vi "Process.vi"(8 "error in":errorcluster, 11 "Plugin in":refnum<class "Sift Stream.lvclass">) -> (0 "error out":errorcluster, 3 "Plugin out":refnum<class "Sift Stream.lvclass">)   [LabVIEW 2024, in "Sift Stream.lvlib" / "Sift Stream.lvclass"]
uses:
  Sift Stream.lvclass
  Sift Stream.lvclass/Sift Stream.ctl
  <vilib>/Utility/error.llb/Error Cluster From Error Code.vi
  <vilib>/ErrorRing/Error Ring.xnode
  <vilib>/Sift/Sift/Sift API/Sift Client.lvclass
  <vilib>/FlexLogger/SDK/PluginSDK.lvlibp/PEFClasses/SDK/Plugin/Plugin.lvclass
  <vilib>/Sift/Sift/Sift Client.lvlib
  C:/Program Files/National Instruments/LabVIEW 2024/vi.lib/FlexLogger/SDK/PluginSDK.lvlibp/PEFClasses/SDK/Plugin/Plugin.lvclass
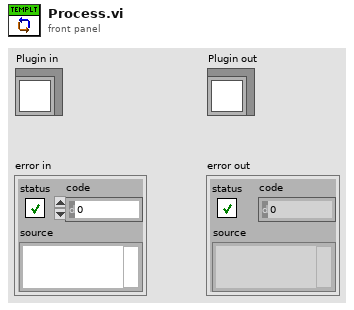
[diagram p1: front panel]
types:
  T1 = typedef "Sift Client.lvlib/Timestamp.ctl" = cluster{"seconds":i64, "nanos":i32}
  T2 = cluster{"Channel Setpoints":dbl[], "Names":string[]}
  T3 = typedef "Sift Stream.lvlib/Sift Stream.lvclass/Sift Stream Parameters.ctl" = cluster{"API gRPC URL":string, "API REST URL":string, "API Key":string, "Asset Name":string, "Data Rate":dbl, "Stream Names":string[], "Sift Client":refnum<class "Sift Client.lvclass">, "Session Error":errorcluster, "Stop Notifier":refnum<notifier>}
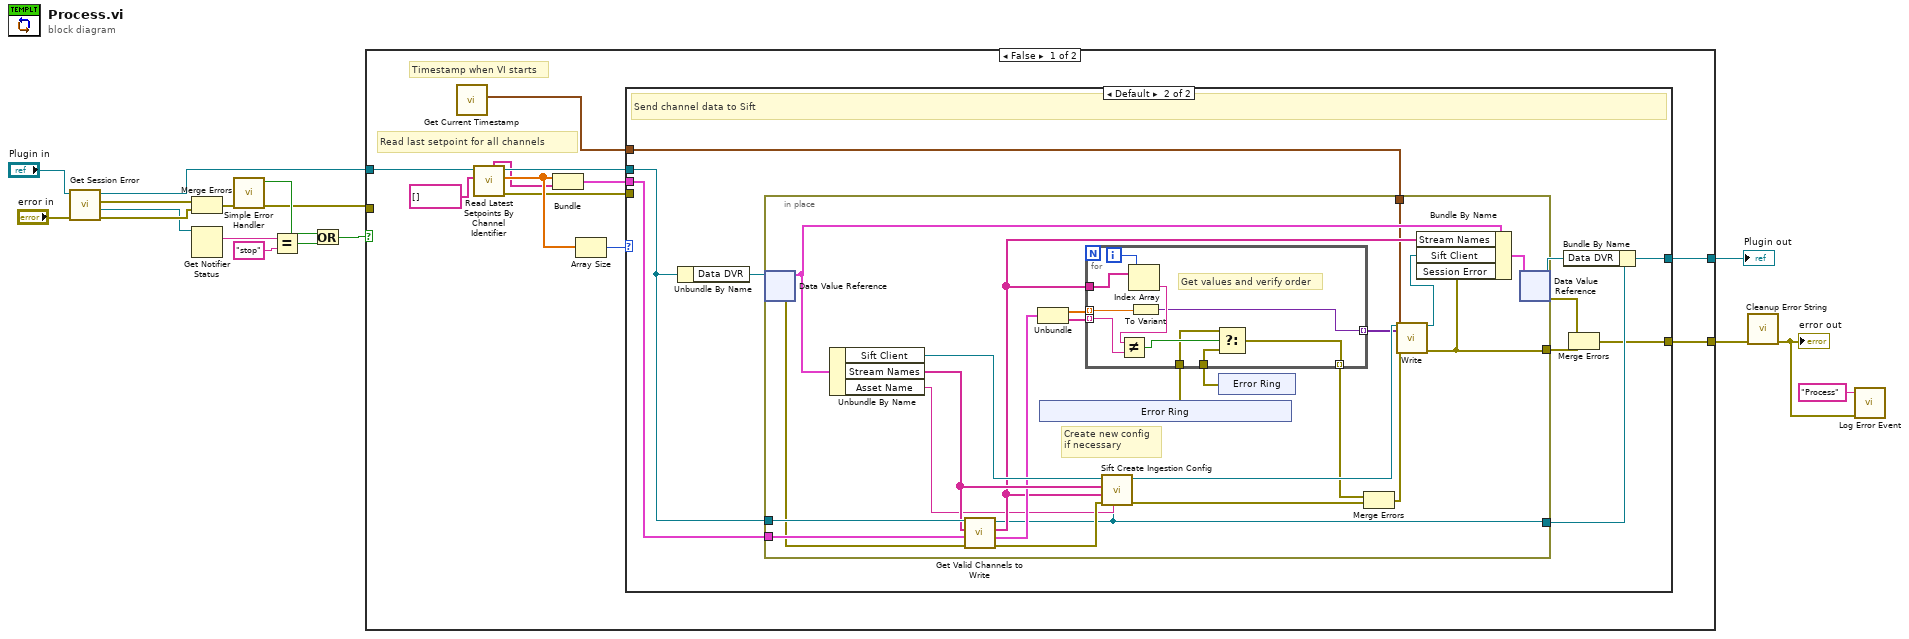
[diagram p0: block diagram]
diagram:
  n1 = call-dynamic "Get Session Error.vi"("error in (no error)"="error in", "Sift Stream in"="Plugin in") -> ("error out"=w10:errorcluster, "Stop Notifier"=w8:refnum<notifier>, "session error"=w11:errorcluster, "Sift Stream out"=w12:refnum<class "Sift Stream.lvclass">)  [unwired: 6 in]
  n2 = Merge Errors(w11, w10) -> (w2:errorcluster)
  n3 = Get Notifier Status(notifier=w8) -> (current notification=w7:string)  [unwired: 1 in, 4 out]
  n4 = call <vilib>:"Simple Error Handler.vi"("error in (no error)"=w2) -> ("error?"=w4:bool, "error out"=w1:errorcluster)  [unwired: 4 in, 3 out]
  n5 = Equal?(x=w7, y="stop") -> (x = y?=w5:bool)
  n6 = Or(x=w4, y=w5) -> (x .or. y?=w3:bool)
  n7 = case shown="False" w3 {
    tunnel: [w27 w82] -> w17
    tunnel: w12 -> [w18 w82]
    tunnel: [w26 w81] -> w16
    tunnel: w1 -> [_ w81]
    frame False {
      # "Timestamp when VI starts"
      # "Read last setpoint for all channels"
      n8 = call <vilib>:"Get Current Timestamp.vi"() -> ("Timestamp"=w20:T1)  [unwired: 11 in]
      n9 = call <vilib>:"Read Latest Setpoints By Channel Identifier.vi"("Unique Channel Identifers (empty = all)"=string[] [], "Plugin in"=w18) -> ("error out"=w22:errorcluster, "Channel Setpoints"=w23:dbl[], "Plugin out"=w21:refnum<class "Sift Stream.lvclass">, "Names"=w19:string[])  [unwired: 6 in]
      n10 = Bundle("Channel Setpoints"=w23, "Names"=w19) -> (w25:T2)  [unwired: 1 in]
      n11 = Array Size(array=w23) -> (size(s)=w28:i32)
      n12 = case shown="Default" w28 {
        tunnel: [w29 w31] -> w26
        tunnel: [w30 w37] -> w27
        tunnel: w21 -> [w30 w35]
        tunnel: w22 -> [w29 _]
        tunnel: w25 -> [_ w36]
        tunnel: w20 -> [_ w33]
        frame 0 {
          # "No channels sending data to the plugin"
        }
        frame Default {
          # "Send channel data to Sift"
          n13 = Unbundle By Name(w35) -> ("Data DVR"=w40:refnum<data-value>)
          n14 = in-place {
            in-place-border: w36 -> [w63]
            in-place-border: w35 -> [w64]
            in-place-border: [w41] -> w34
            in-place-border: w33 -> [w45]
            in-place-border: [w42] -> w32
            # "Create new config\nif necessary"
            n15 = in-place-dvr #1(w40) -> (w62:T3, w61:errorcluster)
            n16 = Unbundle By Name(w62) -> ("Sift Client"=w59:refnum<class "Sift Client.lvclass">, "Stream Names"=w58:string[], "Asset Name"=w43:string)
            n17 = call "Get Valid Channels to Write.vi"("error in (no error)"=w61, "Data to Write In"=w63, "Stream Names In"=w58, "Plugin in"=w64) -> ("error out"=w60:errorcluster, "Data to Write Out"=w54:cluster{dbl[], string[]}, "Stream Names Out"=w51:string[], "Plugin out"=w41:refnum<class "Sift Stream.lvclass">)  [unwired: 4 in]
            n18 = Unbundle(w54) -> (w53:dbl[], w52:string[])
            n19 = xnode "Error Ring"() -> ("error out"=w50:errorcluster)
            n20 = call "Sift Create Ingestion Config.vi"("Asset Name"=w43, "Plugin in"=w41, "error in (no error)"=w60, "New Stream Names"=w51, "Old Stream Names"=w58, "Sift Client in"=w59) -> ("error out"=w47:errorcluster, "Sift Client out"=w56:refnum<class "Sift Client.lvclass">)  [unwired: 4 in]
            n21 = xnode "Error Ring"() -> ("error out"=w49:errorcluster)
            n22 = for {
              tunnel: w53 -> [w80] mode=indexing
              tunnel: w52 -> [w77] mode=indexing
              tunnel: w51 -> [w79]
              tunnel: w50 -> [w74]
              tunnel: w49 -> [w73]
              tunnel: [w72] -> w46 mode=indexing
              tunnel: [w71] -> w44 mode=indexing
              i -> [w78]
              # "Get values and verify order"
              n23 = Index Array(array=w79, index=w78) -> (element=w76:string)
              n24 = Not Equal?(x=w76, y=w77) -> (x != y?=w75:bool)
              n25 = To Variant(anything=w80) -> (Variant=w71:variant)
              n26 = Select(t=w74, s=w75, f=w73) -> (s? t:f=w72:errorcluster)
            }
            n27 = Merge Errors(w46, w47) -> (w48:errorcluster)
            n28 = call-dynamic "Write.vi"("Sift Client in"=w56, "Values"=w44, "Timestamp"=w45, "error in (no error)"=w48) -> ("Sift Client out"=w55:refnum<class "Sift Client.lvclass">, "error out"=w42:errorcluster)  [unwired: 10 in]
            n29 = Bundle By Name(cluster=w62, "Stream Names"=w51, "Sift Client"=w55, "Session Error"=w42) -> (w57:T3)
            n30 = in-place-dvr #1(w57) -> (w38:refnum<data-value>, w39:errorcluster)
          }
          n31 = Bundle By Name(cluster=w34, "Data DVR"=w38) -> (w37:refnum<class "Sift Stream.lvclass">)
          n32 = Merge Errors(w39, w32) -> (w31:errorcluster)
        }
      }
    }
    frame True {
    }
  }
  "Plugin out" <- w17
  n33 = call "Cleanup Error String.vi"("error in (no error)"=w16) -> ("error out"=w15:errorcluster)  [unwired: 10 in]
  "error out" <- w15
  n34 = call "Log Error Event.vi"("error in (no error)"=w15, "Location"="Process") -> ()  [unwired: 10 in]
